vi "ModifyMyAttribute.vi"(0 "reference in":refnum<class "MyG#Class.lvclass">, 2 "increment":dbl, 5 "error in (no error)":errorcluster) -> (14 "reference out":refnum<class "MyG#Class.lvclass">, 19 "error out":errorcluster)   [LabVIEW 2017, in "MyG#Class.lvclass"]
uses:
  MyG#Class.lvclass
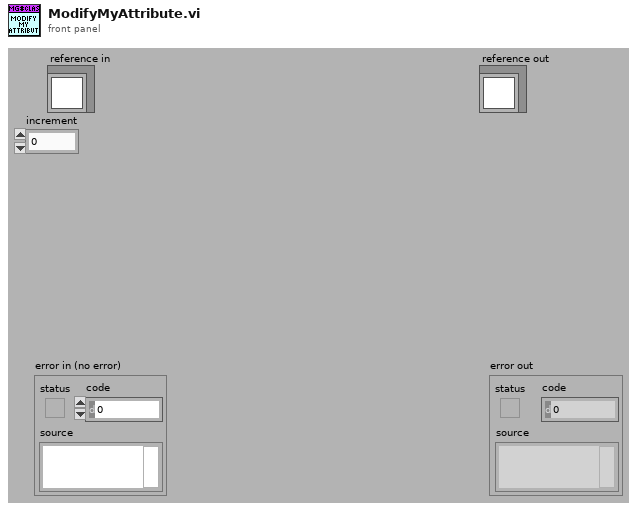
[diagram p1: front panel]
types:
  T1 = typedef "MyG#Class.lvclass/ObjectAttributesRef.ctl" = refnum<data-value>
  T2 = typedef "MyG#Class.lvclass/ObjectAttributes.ctl" = cluster{"MyAttribute":dbl}
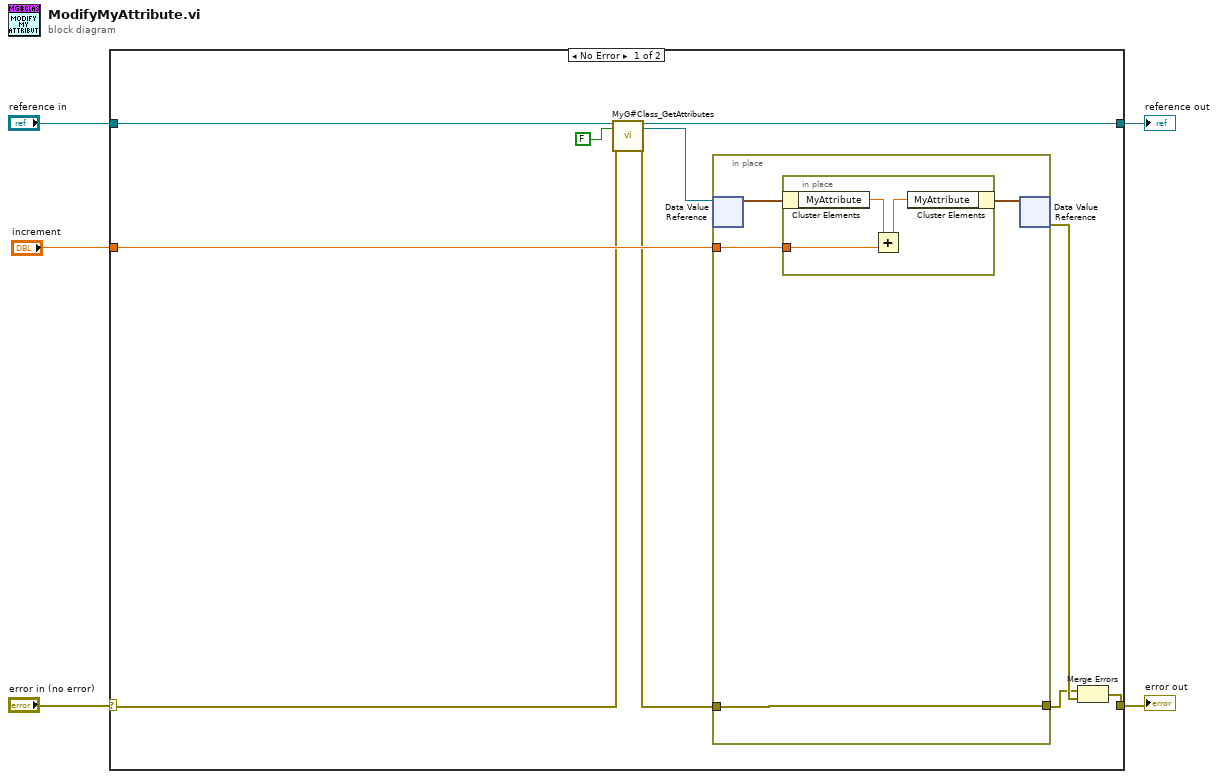
[diagram p0: block diagram]
diagram:
  n1 = case shown="No Error" "error in (no error)" {
    selector: "error in (no error)" -> [w9 w24]
    tunnel: [w15 w24] -> w4
    tunnel: [w10 w23] -> w2
    tunnel: "reference in" -> [w11 w23]
    tunnel: "increment" -> [w12 _]
    frame No Error {
      n2 = call "MyG#Class_GetAttributes.vi"("reference in"=w11, "return data? (T)"=FALSE, "error in (no error)"=w9) -> ("reference out"=w10:refnum<class "MyG#Class.lvclass">, "attributes ref"=w6:T1, "error out"=w8:errorcluster)  [unwired: 13 in, 1 out]
      n3 = in-place {
        in-place-border: w8 -> [w17]
        in-place-border: [w17] -> w13
        in-place-border: w12 -> [w16]
        n4 = in-place-dvr #1(w6) -> (w18:T2)  [unwired: 1 out]
        n5 = in-place {
          in-place-border: w16 -> [w20]
          n6 = in-place-cluster #2(w18) -> ("MyAttribute"=w22:dbl)
          n7 = Add(x=w22, y=w20) -> (x+y=w21:dbl)
          n8 = in-place-cluster #2("MyAttribute"=w21) -> (w19:T2)
        }
        n9 = in-place-dvr #1(w19) -> (w14:errorcluster)  [unwired: 1 out]
      }
      n10 = Merge Errors(w13, w14) -> (w15:errorcluster)
    }
    frame Error {
    }
  }
  "error out" <- w4
  "reference out" <- w2
